vi "Get Node List.vi"(8 "error in (no error)":errorcluster, 11 "CI Deserializer in":refnum<class "CI Deserializer.lvclass">) -> (0 "error out":errorcluster, 1 "Subnodes":string[](array[string]), 2 "Root Node":string)   [LabVIEW 2014, in "CI Deserializer.lvclass"]
uses:
  CI Deserializer.lvclass
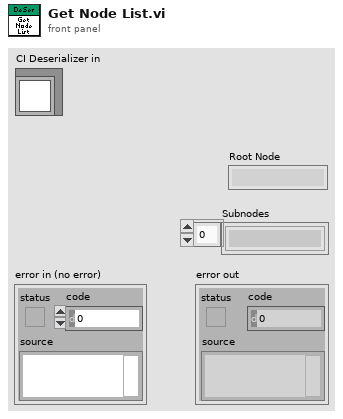
[diagram p1: front panel]
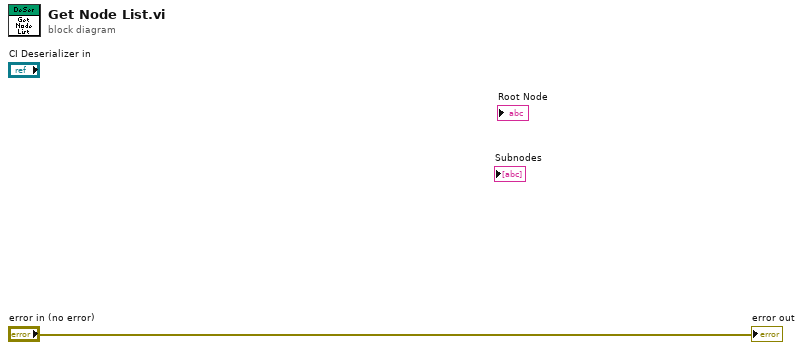
[diagram p0: block diagram]
diagram:
  "error out" <- "error in (no error)"
